vi "Config Key String to DBL Array Group.vi"(7 "Section In":string, 8 "Error In":errorcluster, 10 "Keys In":string[](array[string]), 11 "Ref In":T1) -> (0 "Error Out":errorcluster, 2 "1D DBL Group":cluster{"1D DBL Array Out":dbl[]}[](array[cluster]) {"1D DBL Array Out" format="%#_f"}, 3 "Ref Out":T1)   [LabVIEW 2024]
uses:
  <vilib>/Utility/config.llb/Config Data RefNum.ctl
  <vilib>/Utility/config.llb/NI_LVConfig.lvlib
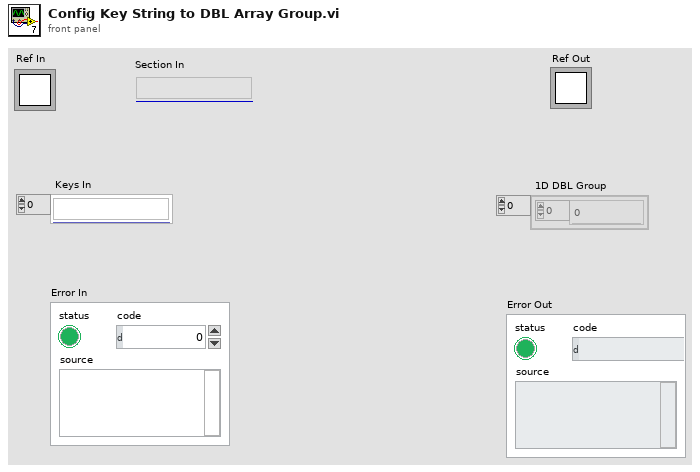
[diagram p1: front panel]
types:
  T1 = typedef "NI_LVConfig.lvlib/Config Data RefNum.ctl" = refnum<k1>
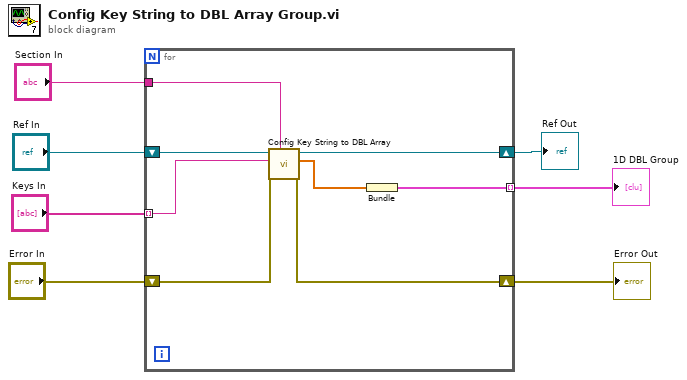
[diagram p0: block diagram]
diagram:
  n1 = for {
    shift-right: [w14] -> w5
    shift-left: "Ref In" -> [w15]
    tunnel: "Section In" -> [w13]
    tunnel: "Keys In" -> [w12] mode=indexing
    tunnel: [w10] -> w3 mode=indexing
    shift-right: [w8] -> w1
    shift-left: "Error In" -> [w9]
    n2 = call "Config Key String to DBL Array.vi"("Section In"=w13, "Error In"=w9, "Key In"=w12, "Ref In"=w15) -> ("Error Out"=w8:errorcluster, "1D DBL Array Out"=w11:dbl[], "Ref Out"=w14:T1)  [unwired: 5 in]
    n3 = Bundle("1D DBL Array Out"=w11) -> (w10:cluster{"1D DBL Array Out":dbl[]})  [unwired: 1 in]
  }
  "Ref Out" <- w5
  "1D DBL Group" <- w3
  "Error Out" <- w1
